vi "svc_Check Frequency Range in Spectrum.vi"(0 "f0":dbl format="%.2f", 5 "df":dbl format="%.2f", 7 "spectrum length":i32, 9 "frequency range":T1 {"stop frequency" format="%.2f"; "start frequency" format="%.2f"}, 11 "error in (no error)":errorcluster) -> (4 "start index":i32, 6 "band length":i32, 8 "f0":dbl format="%.2f", 10 "fmax":dbl format="%.2f", 15 "error out":errorcluster)   [LabVIEW 2017]
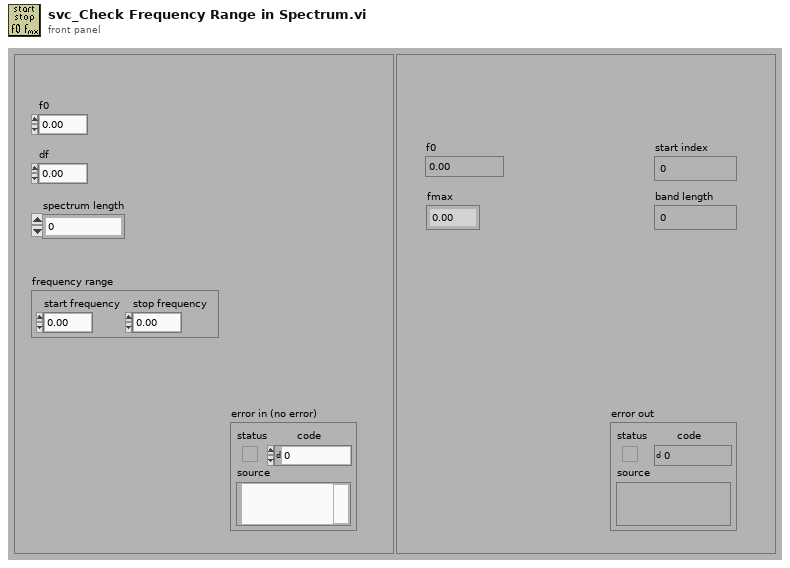
[diagram p1: front panel]
types:
  T1 = cluster{"start frequency":dbl, "stop frequency":dbl}
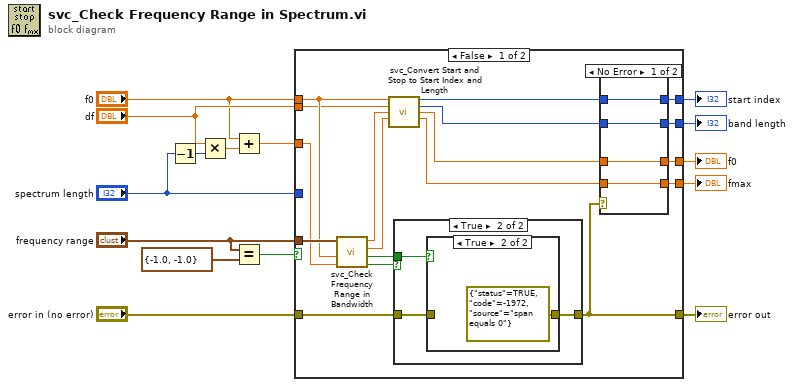
[diagram p0: block diagram]
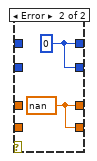
[diagram p2: hidden frame]
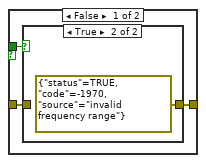
[diagram p3: hidden frame]
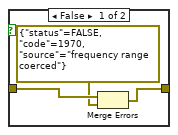
[diagram p4: hidden frame]
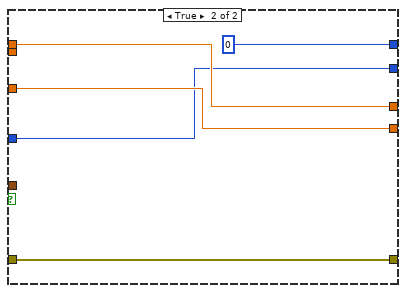
[diagram p6: hidden frame]
diagram:
  n1 = Decrement(x="spectrum length") -> (x-1=w4:i32)
  n2 = Multiply(x="df", y=w4) -> (x*y=w6:dbl)
  n3 = Add(x="f0", y=w6) -> (x+y=w5:dbl)
  n4 = Equal?(x="frequency range", y=T1 {"start frequency"=-1.0, "stop frequency"=-1.0} ("frequency range")) -> (x = y?=w1:bool)
  n5 = case shown="False" w1 {
    tunnel: [w24 w52] -> w15
    tunnel: "error in (no error)" -> [w31 w52]
    tunnel: w5 -> [w27 w55]
    tunnel: [w21 w53] -> w12
    tunnel: [w22 0 ("start index")] -> w13
    tunnel: [w17 w55] -> w11
    tunnel: [w19 w56] -> w10
    tunnel: "df" -> [w25 _]
    tunnel: "f0" -> [w26 w56]
    tunnel: "frequency range" -> [w28 _]
    tunnel: "spectrum length" -> [_ w53]
    frame False {
      n6 = call <vilib>:"svc_Check Frequency Range in Bandwidth.vi"("fmax"=w27, "fmin"=w26, "frequency range"=w28) -> ("start and stop in range"=w33:bool, "zero span"=w32:bool, "stop frequency"=w29:dbl, "start frequency"=w30:dbl)  [unwired: 5 in]
      n7 = call <vilib>:"svc_Convert Start and Stop to Start Index and Length.vi"("f0"=w26, "df"=w25, "start frequency"=w30, "stop frequency"=w29) -> ("start index"=w23:i32, "band length"=w20:i32, "f0 out"=w18:dbl, "fmax out"=w16:dbl)  [unwired: 8 in]
      n8 = case shown="True" w33 {
        tunnel: w31 -> [w40 w48]
        tunnel: [w42 w47] -> w24
        tunnel: w32 -> [w41 w49]
        frame False {
          n9 = case shown="True" w41 {
            tunnel: [w43 errorcluster {"status"=TRUE, "code"=-1970, "source"="invalid frequency range"} ("error in (no error)")] -> w42
            tunnel: w40 -> [w45 _]
            frame False {
              n10 = Merge Errors(w45, errorcluster {"status"=FALSE, "code"=1970, "source"="frequency range coerced"} ("error in (no error)")) -> (w43:errorcluster)
            }
            frame True {
            }
          }
        }
        frame True {
          n11 = case shown="True" w49 {
            tunnel: [w50 errorcluster {"status"=TRUE, "code"=-1972, "source"="span equals 0"} ("error out")] -> w47
            tunnel: w48 -> [w50 _]
            frame False {
            }
            frame True {
            }
          }
        }
      }
      n12 = case shown="No Error" w24 {
        tunnel: w23 -> [w37 _]
        tunnel: [w37 w39] -> w22
        tunnel: [w36 w39] -> w21
        tunnel: w20 -> [w36 _]
        tunnel: [w35 w38] -> w19
        tunnel: w18 -> [w35 _]
        tunnel: [w34 w38] -> w17
        tunnel: w16 -> [w34 _]
        frame No Error {
        }
        frame Error {
          w38 = nan ("f0 out")
          w39 = 0 ("start index")
        }
      }
    }
    frame True {
    }
  }
  "error out" <- w15
  "f0" <- w10
  "start index" <- w13
  "band length" <- w12
  "fmax" <- w11
